vi "Make_Triangle.vi"(1 "N_steps_1":i32 min=0 step=1) -> (0 "TriangleWaveform":dbl[](array[numeric]))   [LabVIEW 2013]
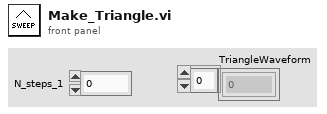
[diagram p1: front panel]
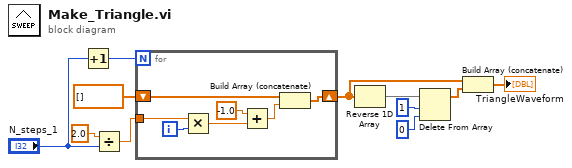
[diagram p0: block diagram]
diagram:
  n1 = Increment(x="N_steps_1") -> (x+1=w8:i32)
  n2 = Divide(x=2.0, y="N_steps_1") -> (x/y=w10:dbl)
  n3 = for {
    N: w8 -> [_]
    tunnel: w10 -> [w16]
    shift-right: [w13] -> w7
    shift-left: dbl[] [] -> [w14]
    i -> [w17]
    n4 = Multiply(x=w16, y=w17) -> (x*y=w15:dbl)
    n5 = Add(x=-1.0, y=w15) -> (x+y=w12:dbl)
    n6 = Build Array (concatenate)(w14, w12) -> (w13:dbl[])
  }
  n7 = Reverse 1D Array(array=w7) -> (reversed array=w5:dbl[])
  n8 = Delete From Array(array=w5, length=1, index=0) -> (array with subset deleted=w4:dbl[])  [unwired: 1 out]
  n9 = Build Array (concatenate)(w7, w4) -> (→"TriangleWaveform":dbl[])
